vi "SwerveJoystickLogic.vi"() -> (2 "Speeds":dbl[](array[numeric]), 3 "Angles":dbl[](array[numeric]))   [LabVIEW 2018]
uses:
  Globals.vi
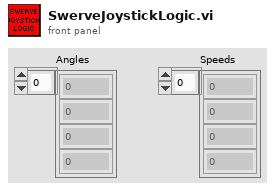
[diagram p1: front panel]
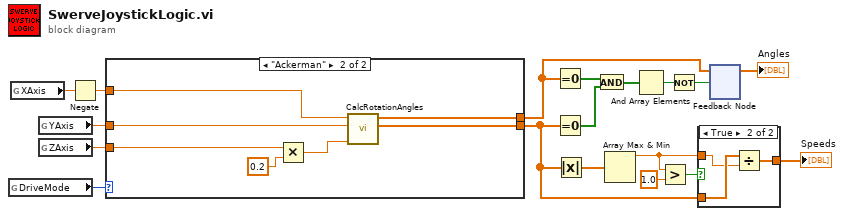
[diagram p0: block diagram]
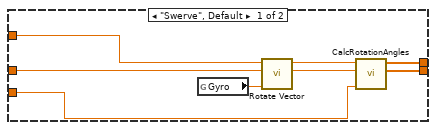
[diagram p3: hidden frame]
diagram:
  n1 = global read "Globals.vi" "DriveMode"() -> (w14:enum16{"Swerve", "Ackerman"})
  n2 = global read "Globals.vi" "XAxis"() -> (w6:dbl)
  n3 = global read "Globals.vi" "YAxis"() -> (w9:dbl)
  n4 = global read "Globals.vi" "ZAxis"() -> (w8:dbl)
  n5 = Negate(x=w6) -> (-x=w5:dbl)
  n6 = case shown="\"Ackerman\"" w14 {
    tunnel: [w26 w30] -> w13
    tunnel: w5 -> [w24 w33]
    tunnel: w9 -> [w23 w32]
    tunnel: w8 -> [w20 w28]
    tunnel: [w25 w31] -> w10
    frame "Swerve", Default {
      n7 = global read "Globals.vi" "Gyro"() -> (w19:dbl)
      n8 = call "Rotate Vector.vi"("Angle"=w19, "Y"=w23, "X"=w24) -> ("Y'"=w21:dbl, "X'"=w22:dbl)  [unwired: 6 in]
      n9 = call "CalcRotationAngles.vi"("ZAxis"=w20, "YAxis"=w21, "XAxis"=w22) -> ("Speeds"=w26:dbl[], "Angles"=w25:dbl[])  [unwired: 7 in]
    }
    frame "Ackerman" {
      n10 = Multiply(x=w28, y=0.2 ("x")) -> (x*y=w29:dbl)
      n11 = call "CalcRotationAngles.vi"("ZAxis"=w29, "YAxis"=w32, "XAxis"=w33) -> ("Speeds"=w30:dbl[], "Angles"=w31:dbl[])  [unwired: 7 in]
    }
  }
  n12 = Equal To 0?(x=w10) -> (x = 0?=w11:bool[])
  n13 = Equal To 0?(x=w13) -> (x = 0?=w4:bool[])
  n14 = Absolute Value(x=w13) -> (abs(x)=w15:dbl[])
  n15 = And(x=w11, y=w4) -> (x .and. y?=w3:bool[])
  n16 = Array Max & Min(array=w15) -> (max value=w16:dbl)  [unwired: 3 out]
  n17 = And Array Elements(Boolean array=w3) -> (logical AND=w2:bool)
  n18 = Greater?(x=w16, y=1.0) -> (0:w18:bool)
  n19 = Not(x=w2) -> (.not. x?=w1:bool)
  n20 = case shown="True" w18 {
    tunnel: w13 -> [w34 w37]
    tunnel: w16 -> [_ w36]
    tunnel: [w34 w35] -> w7
    frame False {
    }
    frame True {
      n21 = Divide(x=w37, y=w36) -> (x/y=w35:dbl[])
    }
  }
  "Speeds" <- w7
  n22 = feedback #1() -> (→"Angles":dbl[])  [unwired: 1 in]
  n23 = feedback-in #1(w10, w1) -> ()
